vi "Ack Stop Notifier.vi"(8 "error in (no error)":errorcluster, 11 "Sift Client in":refnum<class "Sift Client.lvclass">) -> (0 "error out":errorcluster, 3 "Sift Client out":refnum<class "Sift Client.lvclass">)   [LabVIEW 2024, in "Sift Client.lvlib" / "Sift Client.lvclass"]
doc: "Ack the Stop notifier. Used in unit tests."
uses:
  Sift Client.lvclass
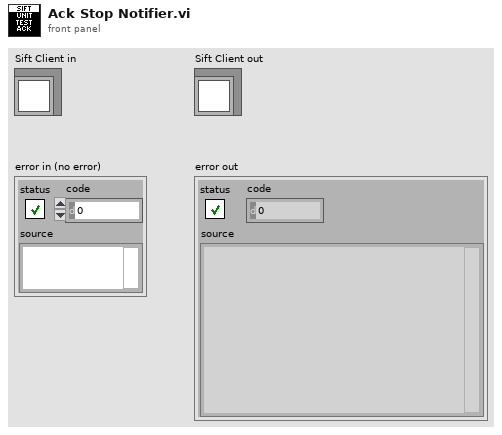
[diagram p1: front panel]
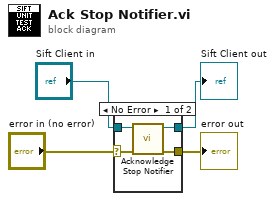
[diagram p0: block diagram]
diagram:
  n1 = case shown="No Error" "error in (no error)" {
    selector: "error in (no error)" -> [w7 w10]
    tunnel: [w6 w10] -> w3
    tunnel: [w5 w9] -> w1
    tunnel: "Sift Client in" -> [w8 w9]
    frame No Error {
      n2 = call-dynamic "Acknowledge Stop Notifier.vi"("error in (no error)"=w7, "Sift Client in"=w8) -> ("error out"=w6:errorcluster, "Sift Client out"=w5:refnum<class "Sift Client.lvclass">)  [unwired: 8 in]
    }
    frame Error {
    }
  }
  "error out" <- w3
  "Sift Client out" <- w1
